vi "ROBOT_DRIVE_PARAMS.vi"() -> (1 "Effective Wheelbase Ft":dbl, 3 "Max Speed Ft/Sec":dbl)   [LabVIEW 2019]
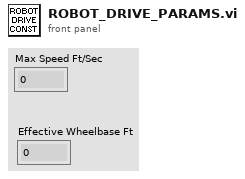
[diagram p1: front panel]
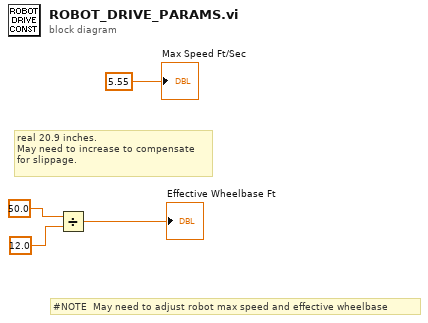
[diagram p0: block diagram]
diagram:
  # "#NOTE  May need to adjust robot max speed and effective wheelbase"
  # "real 20.9 inches.\nMay need to increase to compensate\nfor slippage."
  n1 = Divide(x=50.0, y=12.0) -> (x/y=→"Effective Wheelbase Ft":dbl)
  "Max Speed Ft/Sec" <- 5.55 ("y")
